vi "Autonomous Independent.vi"(8 "Previous Outputs":T2, 9 "Sensor Inputs":T15, 10 "Match Info":T13={"Autonomous Elapsed Seconds"=0.0, "TeleOp Elapsed Seconds"=0.0, "Disabled Elapsed Seconds"=0.0, "Visited Autonomous"=FALSE, "Visited TeleOp"=FALSE, "Visited Disabled"=FALSE, "Autonomous Settings"={"Autonomous Style"=enum."Independent", "VI Refnum"=refnum}}, 11 "Call Context":T14) -> (2 "Auto Commands":T22, 3 "Sensor Inputs (out)":T15)   [LabVIEW 2012]
doc: "This VI is called when autonomous begins, and will automatically be terminated when autonomous ends. You can carry out timed or sensor driven robot movement independently without needing to return to the caller."
uses:
  Inputs_All.ctl
  Flywheel/Sensor_Inputs_FlyWheel.ctl
  tankdrive/Input_Sensors_Drive.ctl
  Conveyor/Sensor_Input_Conveyor.ctl
  Conveyor/Sensor_Input_ConveyorV2.ctl
  Turret/Inputs_Sensors_Turret.ctl
  Inputs_Camera.ctl
  Command_Inputs.ctl
  tankdrive/Input_Commands_Drive.ctl
  Conveyor/Input_Command_Conveyor.ctl
  Turret/Inputs_Commands_Turret.ctl
  Bridge Tipper/Inputs_Tipper.ctl
  Dashboard Controls.ctl
  Roller/Input_Commands_Roller.ctl
  Flywheel/Input_Commands_Flywheel.ctl
  <vilib>/Rock Robotics/WPI/DriverStation/WPI_DriverStationDerivedRobotMode.ctl
  <vilib>/Rock Robotics/WPI/DriverStation/WPI_DriverStationMatch Info.ctl
  Outputs_All.ctl
  Flywheel/Outputs_Flywheel.ctl
  tankdrive/Output_Wheel_Speeds.ctl
  Conveyor/Conveyor_outputs.ctl
  Conveyor/Conveyor module state.ctl
  Conveyor/Conveyor_outputsV2.ctl
  Conveyor/3-Ball-Conveyor_Module_State.ctl
  Conveyor/T_Roller module state.ctl
  Turret/Outputs_Turret.ctl
  Roller/Outputs_Roller.ctl
  Bridge Tipper/Outputs_Tipper.ctl
  <vilib>/Rock Robotics/WPI/DriverStation/WPI_DriverStationRobotMode.ctl
  Robot Global Data.vi
panel:
  in  "Robot Mode":T1
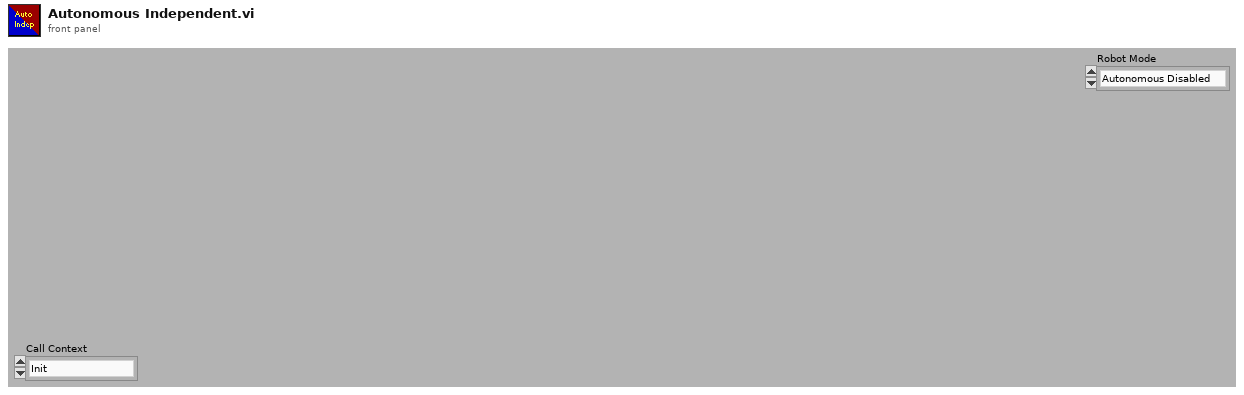
[diagram p1: front panel]
types:
  T1 = typedef "WPI_DriverStationRobotMode.ctl" = enum16{"Autonomous Disabled", "Autonomous Enabled", "Teleop Disabled", "Teleop Enabled", "Timeout", "Finish"}
  T2 = typedef "Outputs_All.ctl" = cluster{"Flywheel Outputs":T3, "Drive Outputs":T4, "Conveyor Outputs":T5, "Conveyor Outputs 2":T7, "Turret Outputs":T10, "Roller Outputs":T11, "Bridge Tipper Outputs":T12}
  T3 = typedef "Outputs_Flywheel.ctl" = cluster{"Wheel Speed":dbl}
  T4 = typedef "Output_Wheel_Speeds.ctl" = cluster{"Front Left Speed":dbl, "Front Right Speed":dbl, "Back Left Speed":dbl, "Back Right Speed":dbl}
  T5 = typedef "Conveyor_outputs.ctl" = cluster{"Bottom Conveyor Speed":dbl, "Top Conveyor Speed":dbl, "Bottom Conveyor State":T6, "Top Conveyor State":T6, "Accepting Balls":bool, "Number of Balls":i32}
  T6 = typedef "Conveyor module state.ctl" = enum16{"No Ball", "Has Ball", "Ball Below Hold", "Ball Above Hold", "Outputting Ball", "Reset"}
  T7 = typedef "Conveyor_outputsV2.ctl" = cluster{"Accepting Balls":bool, "Number of Balls":i32, "Conveyor State":T8, "Top Roller State":T9, "Top Roller":dbl, "Conveyor":dbl}
  T8 = typedef "3-Ball-Conveyor_Module_State.ctl" = enum16{"No Balls", "Collecting Ball", "Holding 1", "Pushing Ball Out", "Holding 2", "Lowering Ball", "Reset", "Disabled"}
  T9 = typedef "T_Roller module state.ctl" = enum16{"Reset", "Disabled", "Waiting for Ball", "Holding", "Ball not far enough", "Ball too far", "Firing"}
  T10 = typedef "Outputs_Turret.ctl" = cluster{"Desired Position":dbl, "Is Reset":bool, "Target In Deadzone":bool}
  T11 = typedef "Outputs_Roller.ctl" = cluster{"Front Roller":dbl}
  T12 = typedef "Outputs_Tipper.ctl" = cluster{"Speed":dbl}
  T13 = typedef "WPI_DriverStationMatch Info.ctl" = cluster{"Autonomous Elapsed Seconds":dbl, "TeleOp Elapsed Seconds":dbl, "Disabled Elapsed Seconds":dbl, "Visited Autonomous":bool, "Visited TeleOp":bool, "Visited Disabled":bool, "Autonomous Settings":cluster{"Autonomous Style":enum16{"Iterative", "Independent"}, "VI Refnum":refnum<vi>}}
  T14 = typedef "WPI_DriverStationDerivedRobotMode.ctl" = enum16{"Init", "Execute", "Stop"}
  T15 = typedef "Inputs_All.ctl" = cluster{"Inputs_FlyWheel":T16, "Drive Inputs":T17, "Conveyor Inputs":T18, "ConveyorV2 Inputs":T19, "Turret Inputs":T20, "Camera Inputs":T21}
  T16 = typedef "Sensor_Inputs_FlyWheel.ctl" = cluster{"Speed":dbl, "Target Distance":dbl}
  T17 = typedef "Input_Sensors_Drive.ctl" = cluster{"Left Front Speed":dbl, "Right Front Speed":dbl, "Left Back Speed":dbl, "Right Back Speed":dbl}
  T18 = typedef "Sensor_Input_Conveyor.ctl" = cluster{"Top Ball Detector Count":i32, "Bottom Ball Detector Count":i32, "Shooter Ball Detector Count":i32}
  T19 = typedef "Sensor_Input_ConveyorV2.ctl" = cluster{"Grab Ball Detector Count":i32, "Bottom Ball Detector Count":i32, "Top In Place Ball Detector Count":i32, "Top Too Far Ball Detector Count":i32, "Top Not Far Enough":i32}
  T20 = typedef "Inputs_Sensors_Turret.ctl" = cluster{"At Minimum Angle":bool, "At Maximum Angle":bool, "Camera Position Offset":dbl, "Found Target?":bool, "Position Encoder":dbl}
  T21 = typedef "Inputs_Camera.ctl" = cluster{"Offset Angle from Perpendicular (degrees)":dbl, "Target Dist":dbl, "Elevation Angle":dbl, "Found Target":bool, "Bounding Rect":cluster{"Left":dbl, "Top":dbl, "Right":dbl, "Bottom":dbl}}
  T22 = typedef "Command_Inputs.ctl" = cluster{"Drive Command Inputs":T23, "Conveyor Command Inputs":T24, "Turret Command Inputs":T25, "Tipper Command Inputs":T26, "Dasboard Controls":T27, "Roller Commands":T28, "Flywheel Commands":T29}
  T23 = typedef "Input_Commands_Drive.ctl" = cluster{"Tank Left Command":dbl, "Tank Right Command":dbl, "Arcade Forward Command":dbl, "Arcade Right Comand":dbl, "Drive Slowly":bool, "Auto-align tipper":bool}
  T24 = typedef "Input_Command_Conveyor.ctl" = cluster{"Shoot a Ball":bool, "Reset":bool, "Enable Conveyor":bool}
  T25 = typedef "Inputs_Commands_Turret.ctl" = cluster{"Reset Turret":bool, "User Position Change Command":dbl, "Aim with camera":bool}
  T26 = typedef "Inputs_Tipper.ctl" = cluster{"Tipper Comand":dbl}
  T27 = typedef "Dashboard Controls.ctl" = cluster{"Joystick Right/Left":dbl, "Joystick Up/Down":dbl, "Use top camera":bool}
  T28 = typedef "Input_Commands_Roller.ctl" = cluster{"Enable Front Roller":bool}
  T29 = typedef "Input_Commands_Flywheel.ctl" = cluster{"Key Mode":bool, "Layup Mode":bool, "Flywheel Speed Offset":dbl, "Distance Mode":bool, "Lob Mode":bool, "Reset":bool, "Reverse (slow)":bool}
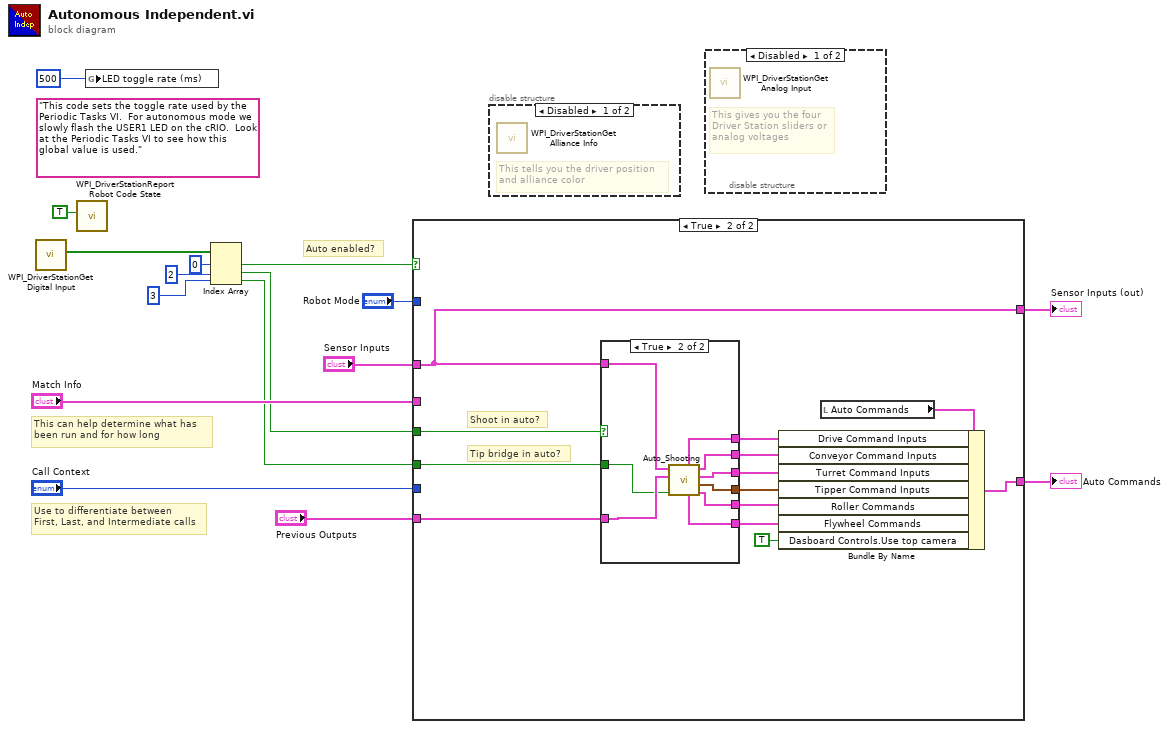
[diagram p0: block diagram]
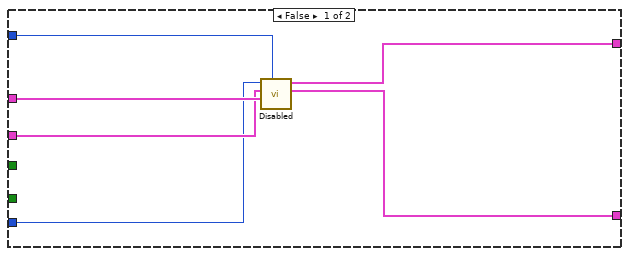
[diagram p2: hidden frame]
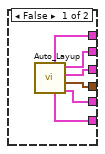
[diagram p3: hidden frame]
diagram:
  (unwired) "This code sets the toggle rate used by the Periodic Tasks VI.  For autonomous mode we slowly flash the USER1 LED on the cRIO.  Look at the Periodic Tasks VI to see how this global value is used."
  # "Use to differentiate between\nFirst, Last, and Intermediate calls"
  # "This can help determine what has\nbeen run and for how long"
  # "Auto enabled?"
  n1 = call <vilib>:"WPI_DriverStationGet Digital Input.vi"() -> ("Driver Station Digital Input (1-8)"=w16:bool[])  [unwired: 11 out]
  n2 = call <vilib>:"WPI_DriverStationReport Robot Code State.vi"("Autonomous"=TRUE) -> ()  [unwired: 10 in, 1 out]
  n3 = global write "Robot Global Data.vi" "LED toggle rate (ms)"(u32 500 ("LED ms toggle rate")) -> ()
  n4 = Index Array(array=w16, index #1=0 ("index"), index #2=2 ("index"), index #3=3 ("index")) -> (element #1=w12:bool, element #2=w4:bool, element #3=w1:bool)
  n5 = case shown="True" w12 {
    tunnel: "Sensor Inputs" -> [w22 w33]
    tunnel: [w21 w33] -> w10
    tunnel: [w20 w34] -> w9
    tunnel: "Match Info" -> [w19 _]
    tunnel: "Call Context" -> [w18 _]
    tunnel: "Previous Outputs" -> [_ w32]
    tunnel: "Robot Mode" -> [w17 _]
    tunnel: w4 -> [_ w24]
    tunnel: w1 -> [_ w23]
    frame False {
      n6 = call "Disabled.vi"("Robot Mode"=w17, "Sensor Inputs (in)"=w22, "Match Info"=w19, "Call Context"=w18) -> ("Disabled Commands"=w20:T22, "Sensor Inputs (out)"=w21:T15)  [unwired: 6 in]
    }
    frame True {
      # "Tip bridge in auto?"
      # "Shoot in auto?"
      n7 = case shown="True" w24 {
        tunnel: w33 -> [_ w50]
        tunnel: w32 -> [_ w49]
        tunnel: [w39 w48] -> w31
        tunnel: [w40 w47] -> w30
        tunnel: [w41 w46] -> w29
        tunnel: [w38 w45] -> w28
        tunnel: [w37 w44] -> w27
        tunnel: [w36 w43] -> w26
        tunnel: w23 -> [_ w42]
        frame False {
          n8 = call "Auto_Layup.vi"() -> ("Roller Commands"=w37:T28, "Tipper Command Inputs"=w38:T26, "Turret Command Inputs"=w39:T25, "Conveyor Command Inputs"=w40:T24, "Flywheel Commands"=w36:T29, "Drive Command Inputs"=w41:T23)  [unwired: 6 in]
        }
        frame True {
          n9 = call "Auto_Shooting.vi"("Tip Bridge in auto"=w42, "Previous Outputs"=w49, "Sensor Inputs"=w50) -> ("Roller Commands"=w44:T28, "Tipper Command Inputs"=w45:T26, "Turret Command Inputs"=w48:T25, "Conveyor Command Inputs"=w47:T24, "Flywheel Commands"=w43:T29, "Drive Command Inputs"=w46:T23)  [unwired: 3 in]
        }
      }
      n10 = local read "Auto Commands"() -> (w35:T22)
      n11 = Bundle By Name(cluster=w35, "Drive Command Inputs"=w29, "Conveyor Command Inputs"=w30, "Turret Command Inputs"=w31, "Tipper Command Inputs"=w28, "Roller Commands"=w27, "Flywheel Commands"=w26, "Dasboard Controls.Use top camera"=TRUE) -> (w34:T22)
    }
  }
  "Auto Commands" <- w9
  "Sensor Inputs (out)" <- w10
  n12 = disable-structure shown="Disabled" {
    frame Disabled {
      # "This tells you the driver position\nand alliance color"
      n13 = call <vilib>:"WPI_DriverStationGet Alliance Info.vi"() -> ()  [unwired: 12 out]
    }
    frame Enabled {
    }
  }
  n14 = disable-structure shown="Disabled" {
    frame Disabled {
      # "This gives you the four\nDriver Station sliders or\nanalog voltages"
      n15 = call <vilib>:"WPI_DriverStationGet Analog Input.vi"() -> ()  [unwired: 12 out]
    }
    frame Enabled {
    }
  }
